vi "ALTS-2015 Enqueue Rerun Task State.vi"(8 "error in (no error)":errorcluster, 11 "Stations to Rerun In":T1[](array[typedef])) -> (0 "error out":errorcluster, 3 "Stations to Rerun Out":T1[](array[typedef]))   [LabVIEW 2013]
uses:
  Controls/ALTS-2015 Station Cluster.ctl
  Controls/ALTS-2015 LV2GBL Station Info Options.ctl
  Controls/ALTS-2015 Ring Indicator Enum.ctl
  Controls/ALTS-2015 Status Ring Indicator.ctl
  Controls/ALTS-2015 Robot FIFO Queue Options.ctl
  Controls/ALTS-2015 Robot Tasks.ctl
  Controls/ALTS-2015 Serial Details.ctl
  Controls/ALTS-2015 Serial DB Details.ctl
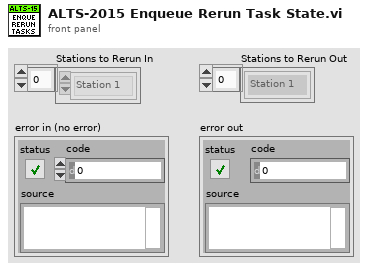
[diagram p1: front panel]
types:
  T1 = typedef "ALTS-2015 Station Cluster.ctl" = enum16{"Station 1", "Station 2", "Station 3", "Station 4"}
  T2 = typedef "ALTS-2015 Status Ring Indicator.ctl" = u16
  T3 = typedef "ALTS-2015 Ring Indicator Enum.ctl" = enum16{"Idle", "Test Running", "Unit Clamped", "Unit not Clamped", "Pass", "Fail"}
  T4 = typedef "ALTS-2015 LV2GBL Station Info Options.ctl" = enum16{"Init", "Read", "Read All", "Write Sensor ID", "Write  Work Order", "Write Serial Number", "Write Test Data", "Write Station Status", "Write Station Occupancy", "Write Station Test Type", "Write Rerun", "Write Load Decision", "Write Robot Action", "Clear All", "Clear Test Result"}
  T5 = typedef "ALTS-2015 Robot Tasks.ctl" = enum16{"Load", "Unload", "Rerun", "Invalid Serial"}
  T6 = typedef "ALTS-2015 Robot FIFO Queue Options.ctl" = enum16{"Init", "Enqueue", "Dequeue", "Get Queue Elements", "Flush", "Destroy"}
  T7 = typedef "ALTS-2015 Station Details.ctl" = cluster{"Station Number":string, "Work Order Number":string, "Sensor Name":string, "Pressure (PSI)":string, "Flow (SCCM)":string, "Test Time ":string, "Test Result":string, "Serial Number":string, "Station Status":T2, "SW assigned UUT":bool, "Rerun Count":i32, "Test Type":i32, "Load Decision":i32, "Robot Action":T8}
  T8 = typedef "ALTS-2015 Robot Actions.ctl" = enum16{"Loading...", "Unloading...", "Reruning...", "No Action"}
  T9 = typedef "ALTS-2015 Serial Details.ctl" = cluster{"Robot Task":T5, "Serial No":string, "New Serial?":bool, "Station # Unload":T1, "Last Test Result":bool, "Rerun?":bool, "Station # Rerun":T1, "Invalid Serial?":bool, "Serial Details":T10}
  T10 = typedef "ALTS-2015 Serial DB Details.ctl" = cluster{"Adapter Plate Size":i32, "Air Leak Test Type ":i32, "Displacement Size":i32, "Flange Size":i32, "Height":i32, "Load Decision":i32, "Cart Insert":i32}
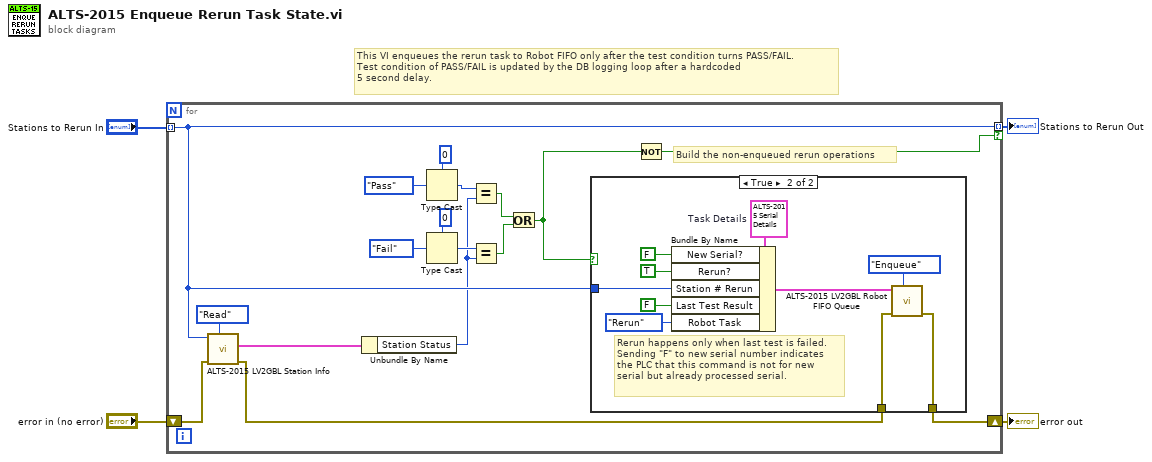
[diagram p0: block diagram]
diagram:
  # "This VI enqueues the rerun task to Robot FIFO only after the test condition turns PASS/FAIL.\nTest condition of PASS/FAIL is updated by the DB logging loop after a hardcoded\n5 second delay."
  n1 = for {
    tunnel: "Stations to Rerun In" -> [w17] mode=indexing
    shift-right: [w21] -> w2
    shift-left: "error in (no error)" -> [w19]
    tunnel: [w17] -> w4 mode=indexing if=w5
    # "Build the non-enqueued rerun operations"
    n2 = call "ALTS-2015 LV2GBL Station Info.vi"("Options"=ALTS-2015_LV2GBL_Station_Info_Options."Read", "error in"=w19, "Station Cluster"=w17) -> ("error out"=w18:errorcluster, "Station Details"=w15:T7)  [unwired: 6 in, 1 out]
    n3 = Unbundle By Name(w15) -> ("Station Status"=w7:T2)
    n4 = Type Cast(type=T2 0 ("Station Status"), x=ALTS-2015_Ring_Indicator_Enum."Pass" ("Ring Indicator Options")) -> (*(type *) &x=w10:T2)
    n5 = Type Cast(type=T2 0 ("Station Status"), x=ALTS-2015_Ring_Indicator_Enum."Fail" ("Ring Indicator Options")) -> (*(type *) &x=w14:T2)
    n6 = Equal?(x=w10, y=w7) -> (x = y?=w6:bool)
    n7 = Equal?(x=w14, y=w7) -> (x = y?=w13:bool)
    n8 = Or(x=w6, y=w13) -> (x .or. y?=w12:bool)
    n9 = case shown="True" w12 {
      tunnel: w18 -> [w22 w32]
      tunnel: [w22 w27] -> w21
      tunnel: w17 -> [_ w25]
      frame False {
      }
      frame True {
        w31 = T9 {"Robot Task"=enum."Load", "Serial No"="", "New Serial?"=FALSE, "Station # Unload"=enum."Station 1", "Last Test Result"=FALSE, "Rerun?"=FALSE, "Station # Rerun"=enum."Station 1", "Invalid Serial?"=FALSE, "Serial Details"={"Adapter Plate Size"=0, "Air Leak Test Type "=0, "Displacement Size"=0, "Flange Size"=0, "Height"=0, "Load Decision"=0, "Cart Insert"=0}}  # Task Details
        # "Rerun happens only when last test is failed.\nSending \"F\" to new serial number indicates\nthe PLC that this command is not for new\nserial but already processed serial."
        n10 = Bundle By Name(cluster=w31, "New Serial?"=FALSE ("New Part?"), "Rerun?"=TRUE, "Station # Rerun"=w25, "Last Test Result"=FALSE, "Robot Task"=ALTS-2015_Robot_Tasks."Rerun") -> (w28:T9)
        n11 = call "ALTS-2015 LV2GBL Robot FIFO Queue.vi"("Options"=ALTS-2015_Robot_FIFO_Queue_Options."Enqueue" ("Enum"), "error in (no error)"=w32, "Task Details In"=w28) -> ("error out"=w27:errorcluster)  [unwired: 4 in, 4 out]
      }
    }
    n12 = Not(x=w12) -> (.not. x?=w5:bool)
  }
  "Stations to Rerun Out" <- w4
  "error out" <- w2
